vi "Write Startup Views.vi"(7 "Popup Title":string, 9 "View Labels (optional)":string[](array[string]), 10 "Viewables":refnum<class "IViewable.lvclass">[](array[class]), 11 "Popup ViewManager in":refnum<class "Popup ViewManager.lvclass">) -> (3 "Popup ViewManager out":refnum<class "Popup ViewManager.lvclass">)   [LabVIEW 2020, in "Popup ViewManager.lvlib" / "Popup ViewManager.lvclass"]
uses:
  <vilib>/gpm_packages/@cs/popup-viewmanager/Source/Popup ViewManager/Popup ViewManager.lvclass
  <vilib>/gpm_packages/@cs/mva-viewable/Source/IViewable/IViewable/IViewable.lvclass
  <vilib>/gpm_packages/@cs/popup-viewmanager/Source/Popup ViewManager/Popup ViewManager.lvclass/Popup ViewManager.ctl
  <vilib>/gpm_packages/@cs/popup-viewmanager/Source/Popup ViewManager Messages/Launch Nested Views Msg/Launch Nested Views Msg.lvclass
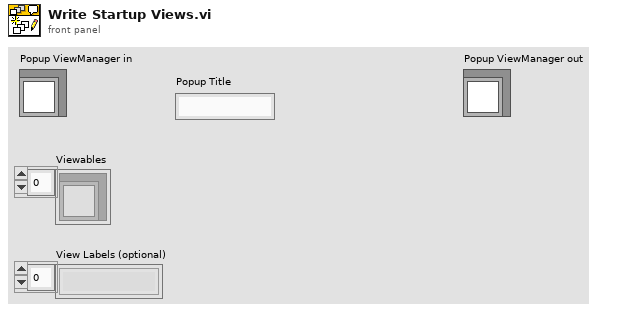
[diagram p1: front panel]
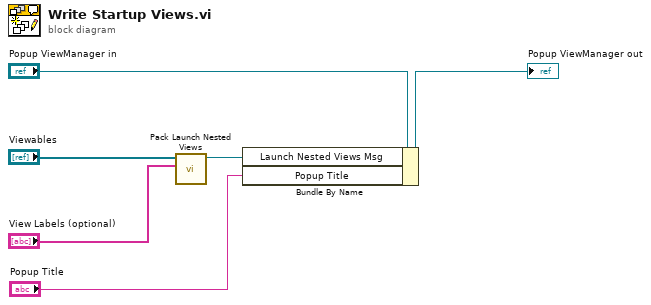
[diagram p0: block diagram]
diagram:
  n1 = call <vilib>:"Pack Launch Nested Views.vi"("View Labels (optional)"="View Labels (optional)", "Viewables"="Viewables") -> ("Launch Nested Views Msg"=w2:refnum<class "Launch Nested Views Msg.lvclass">)  [unwired: 9 in]
  n2 = Bundle By Name(cluster="Popup ViewManager in", "Launch Nested Views Msg"=w2, "Popup Title"="Popup Title") -> (→"Popup ViewManager out":refnum<class "Popup ViewManager.lvclass">)
